vi "OAT Get Vector Reference.vi"   [LabVIEW 2017, in "SoundVib_RefDataProcess.lvlib"]
doc: "Computes the vector references of the specified orders from the slow-roll vibration signals. Use the vector references to compensate shaft bow or runout errors. Wire data to the <B>scaled signal [EU]</B> input to determine the polymorphic instance to use or manually select the instance."
uses:
  <vilib>/addons/Sound and Vibration/Order Analysis/Referece Data Processing/SoundVib_RefDataProcess.lvlib
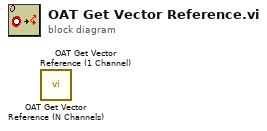
[diagram p0: block diagram]
diagram:
  n1 = call <vilib>:"OAT Get Vector Reference (N Channels).vi"() -> ()  [unwired: 14 in, 2 out]
  n2 = call <vilib>:"OAT Get Vector Reference (1 Channel).vi"() -> ()  [unwired: 14 in, 2 out]
